vi "PWM_Test.vi"() -> ()   [LabVIEW 2020]
uses:
  LabVIEW 2020 Toolkits/VI Server Toolkit/VI Server_TypeDefs/VI Server_RefsCluster.ctl
  LabVIEW 2020 Toolkits/VI Server Toolkit/VI Server Libraries/VI Server_GetControl.llb/VI Server_DBL_Get.vi
  DAQNavi/LabviewDriver/VI/DAQNavi Polymorphic VI/create/DAQNavi Create Channel(CO-Pulse Width).vi
panel:
  in  "VI Server.RefsCluster":T1
  in  "PWM.Ch1.Start":bool caption="Counter.Start"
  in  "PWM.Ch1.Period.Hi":dbl caption="Period: Hi" format="%#_g ms"
  in  "PWM.Ch1.Period.Lo":dbl caption="Period: Lo" format="%#_g ms"
  in  "Stop Button":bool
  out "error out":errorcluster
  in  "error in (no error)":errorcluster
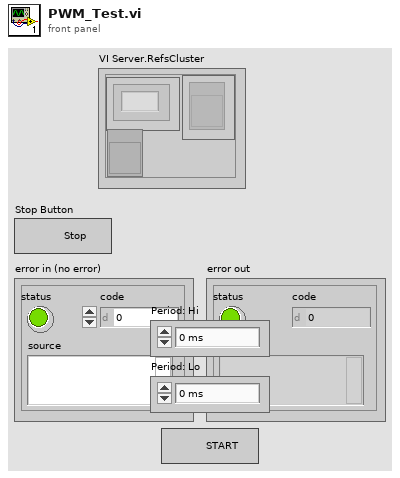
[diagram p1: front panel]
types:
  T1 = typedef "VI Server_RefsCluster.ctl" = cluster{"Labels":string[], "Refs":refnum<vi>[], "VI Ref":refnum<vi>}
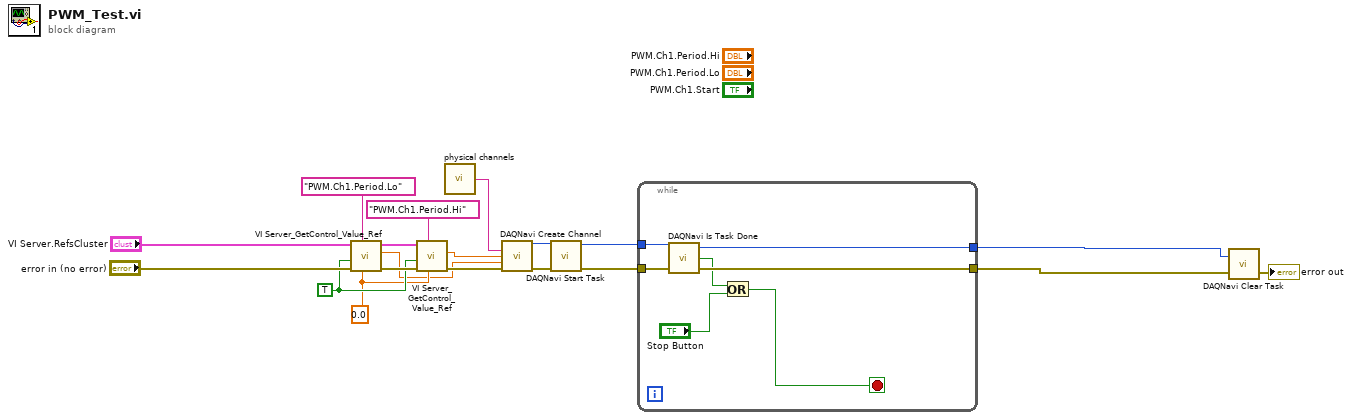
[diagram p0: block diagram]
diagram:
  w4 = 0.0
  w7 = TRUE ("SingleInstance")
  n1 = call-poly "VI Server_GetControl_Value_Ref.vi"("DataType"=w4, "Control.Label"="PWM.Ch1.Period.Lo", "error in"="error in (no error)", "SingleInstance"=w7, "VI Server.RefsCluster"="VI Server.RefsCluster") -> ("error out"=w11:errorcluster, "Value"=w1:dbl, "VI Server.RefsCluster.DUP"=w6:T1)  [unwired: 3 in, 1 out]
  n2 = call-poly "VI Server_GetControl_Value_Ref.vi"("DataType"=w4, "Control.Label"="PWM.Ch1.Period.Hi", "error in"=w11, "SingleInstance"=w7, "VI Server.RefsCluster"=w6) -> ("error out"=w9:errorcluster, "Value"=w2:dbl)  [unwired: 3 in, 2 out]
  n3 = call "physical channels"() -> ("property value"=w18:string)  [unwired: 1 out]
  n4 = call-poly "DAQNavi Create Channel.vi"("physical channels"=w18, "high period"=w2, "low period"=w1, "error in (no error)"=w9) -> ("task out"=w17:i32, "error out"=w16:errorcluster)  [unwired: 1 in, 9 out]
  n5 = call "DAQNavi Start Task.vi"("error in (no error)"=w16, "task in"=w17) -> ("error out"=w15:errorcluster, "task out"=w14:i32)  [unwired: 8 out]
  n6 = while {
    tunnel: w15 -> [w26]
    tunnel: w14 -> [w25]
    tunnel: [w24] -> w13
    tunnel: [w23] -> w12
    stop <- w20 stop-if-true
    n7 = call "DAQNavi Is Task Done.vi"("error in (no error)"=w26, "task in"=w25) -> ("error out"=w24:errorcluster, "isTaskDone"=w22:bool, "task out"=w23:i32)  [unwired: 1 out]
    n8 = Or(x=w22, y="Stop Button") -> (x .or. y?=w20:bool)
  }
  n9 = call "DAQNavi Clear Task.vi"("error in (no error)"=w13, "task in"=w12) -> ("error out"=→"error out":errorcluster)  [unwired: 1 out]
